vi "Shutdown Calibrator.vi"(8 "error in":errorcluster, 11 "COM Port":string) -> (0 "error out":errorcluster)   [LabVIEW 2013]
doc: "Fluke 5080.lvlib:Error Query.vi\nInstrument reports:\n1\n0,\"No Error {REM}\"\n\n\n\nComplete call chain:\n Fluke 5080.lvlib:Error Query.vi\n Fluke 5080.lvlib:Configure Output.vi\n Shutdown Calibrator.vi\n Shutdown Calibrator.vi.ProxyCaller\nLabVIEW: Instrument error query failure.\n\n\n-1074000000; User-defined error code.\n\n\nStep 'Shutdown Calibrator' of sequence 'Full Scale Voltage Calibration' in 'Snap-On Tablet Scope Test.seq'"
uses:
  <instrlib>/Fluke 5080/Fluke 5080.lvlib
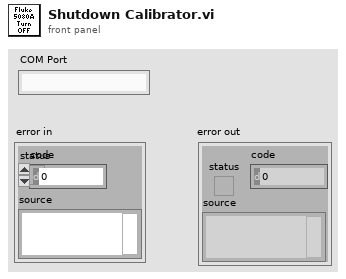
[diagram p1: front panel]
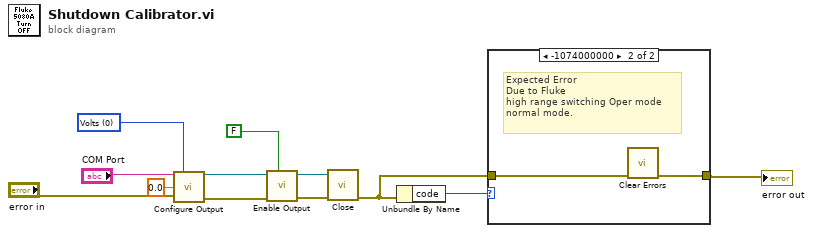
[diagram p0: block diagram]
diagram:
  w6 = 0 items=["Volts", "dBm"] ("Voltage Unit (0: Volts)")
  n1 = call <instrlib>:"Configure Output.vi"("VISA resource name"="COM Port", "Voltage Unit (0: Volts)"=w6, "Primary Voltage (5.0)"=0.0, "error in (no error)"="error in") -> ("VISA resource name out"=w8:refnum<visa-resource-name>, "error out"=w9:errorcluster)  [unwired: 10 in]
  n2 = call <instrlib>:"Enable Output.vi"("Output Enabled (T: Enable)"=FALSE, "error in (no error)"=w9, "VISA resource name"=w8) -> ("error out"=w4:errorcluster, "VISA resource name out"=w3:refnum<visa-resource-name>)  [unwired: 7 out]
  n3 = call <instrlib>:"Close.vi"("error in (no error)"=w4, "VISA resource name"=w3) -> ("error out"=w2:errorcluster)  [unwired: 9 in]
  n4 = Unbundle By Name(w2) -> ("code"=w11:i32)
  n5 = case shown="-1074000000" w11 {
    tunnel: w2 -> [w13 w15]
    tunnel: [w13 w14] -> w1
    frame 0, Default {
    }
    frame -1074000000 {
      # "Expected Error\nDue to Fluke\nhigh range switching Oper mode\nnormal mode."
      n6 = call <vilib>:"Clear Errors.vi"("error in (no error)"=w15) -> ("error out"=w14:errorcluster)  [unwired: 6 in]
    }
  }
  "error out" <- w1
